vi "hmi-application.vi"() -> ()   [LabVIEW 2017]
doc: "Demonstrates how to write and receive CAN frames via the Network Interface on the same port. \n\nTo write and receive frames via the Network Interface:\n- select the CAN Network Interface (i.e. CAN0, CAN1, etc.)\n- select the Baud Rate\n- run the VI\n- press the write button to write frames to the can bus\n\nEnable RTR Button to send a Remote Transmission Request or to simply send an empty Frame to request an Answer Frame from a connected device.\n\nEnable Extended Button to write extended Identifier Format. This is done by setting the 30th bit to enable extended format with the driver."
uses:
  <vilib>/nican/nican.llb/ncNetAttr.ctl
panel:
  in  "Tab Control":enum32{"Program", "Settings"}(tab)
  in  "shutdown":bool
  in  "IND1":bool
  in  "IND2":bool
  in  "interface":string(combo)="CAN0" caption="Interface"
  # "PRESS AND HOLD"
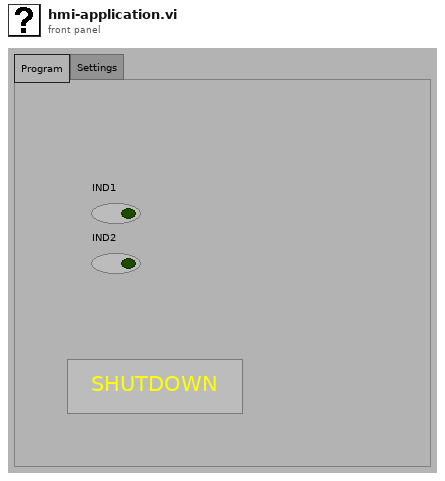
[diagram p1: front panel]
types:
  T1 = typedef "ncNetAttr.ctl" = cluster{"Start On Open":enum32{"FALSE", "TRUE"}, "Baud Rate":u32, "Read Queue Length":u32, "Write Queue Length":u32, "Standard Comparator":u32, "Standard Mask":u32, "Extended Comparator":u32, "Extended Mask":u32}
  T2 = typedef "xobjhandle.ctl" = u32
  T3 = typedef "CanFrameTimed.ctl" = cluster{"Timestamp":dbl, "ArbitrationId":u32, "IsRemote":u8, "DataLength":u8, "Data":u8[]}
  T4 = cluster{dbl, u32, "IsRemote":u8, "DataLength":u8, u8[]}
  T5 = cluster{dbl, u32, "IsRemote":u8, "DataLength":u8, u8[]}[]
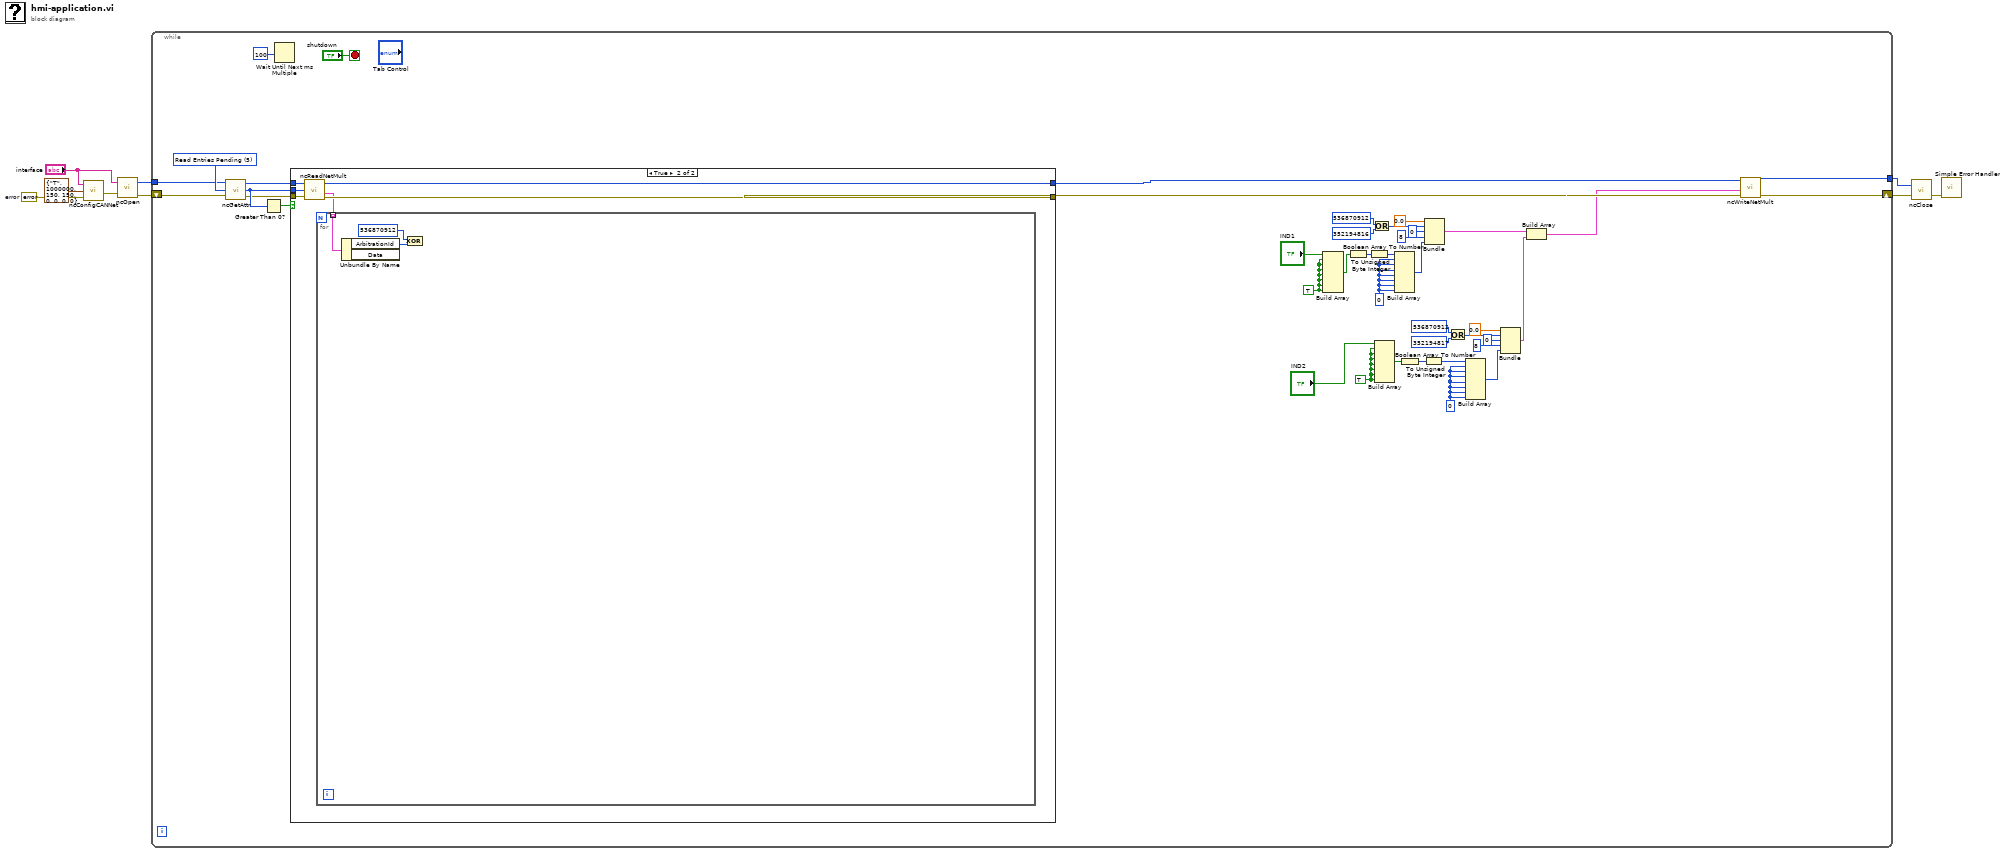
[diagram p0: block diagram]
diagram:
  w5 = errorcluster {"status"=FALSE, "code"=0, "source"=""}  # error
  n1 = call <vilib>:"ncConfigCANNet.vi"("Error in"=w5, "CAN Network Interface Config"=T1 {"Start On Open"=enum."TRUE", "Baud Rate"=1000000, "Read Queue Length"=150, "Write Queue Length"=150, "Standard Comparator"=0, "Standard Mask"=0, "Extended Comparator"=0, "Extended Mask"=0}, "ObjName"="interface") -> ("Error out"=w6:errorcluster)  [unwired: 2 in]
  n2 = call <vilib>:"ncOpen.vi"("Error in"=w6, "ObjName"="interface") -> ("Error out"=w9:errorcluster, "ObjHandle out"=w7:T2)
  n3 = while {
    tunnel: w7 -> [w40]
    tunnel: [w50] -> w2
    shift-right: [w51] -> w1
    shift-left: w9 -> [w39]
    stop <- "shutdown" stop-if-true
    w18 = TRUE ("element")
    w20 = TRUE ("element")
    w23 = u8 0
    w31 = u8 0
    w43 = u32 5 items=["(reserved)", "Protocol Version", "Software Version", "Object State", "(reserved)", "Read Entries Pending", "Write Entries Pending", "ReadMult Size for Notification", "Listen Only?", "Self Reception?", "Transmit Error Counter", "Receive Error Counter", "Single Shot Transmit?", "Series 2 Filter Mode", "Series 2 Mask", "Series 2 Comparator", "Serial Number", "Form Factor", "Series", "Transceiver Type", "Interface Number", "Series 2 Error/Arb Capture", "Transceiver Mode", "Transceiver External Outputs", "Transceiver External Inputs", "Start Trigger Behavior", "Log Comm Warnings", "User RTSI Frame", "Transmit Mode", "Log Start Trigger?", "Timestamp Format", "Master Timebase Rate", "Virtual Bus Timing"] ("AttrId")
    n4 = call <vilib>:"ncGetAttr.vi"("Error in"=w39, "AttrId"=w43, "ObjHandle in"=w40) -> ("Error out"=w44:errorcluster, "AttrValue"=w47:u32, "ObjHandle out"=w45:T2)
    n5 = Greater Than 0?(x=w47) -> (x > 0?=w46:bool)
    n6 = Wait Until Next ms Multiple(millisecond multiple=u32 100) -> ()  [unwired: 1 out]
    n7 = case shown="True" w46 {
      tunnel: [w52 w59] -> w41
      tunnel: [w53 w58] -> w42
      tunnel: w47 -> [_ w57]
      tunnel: w44 -> [w52 w56]
      tunnel: w45 -> [w53 w55]
      frame False {
      }
      frame True {
        n8 = call <vilib>:"ncReadNetMult.vi"("ObjHandle in"=w55, "Requested Number of Frames"=w57, "Error in"=w56) -> ("ObjHandle out"=w58:T2, "Data"=w54:T3[], "Error out"=w59:errorcluster)  [unwired: 1 out]
        n9 = for {
          tunnel: w54 -> [w62] mode=indexing
          n10 = Unbundle By Name(w62) -> ("ArbitrationId"=w60:u32)  [unwired: 1 out]
          n11 = Exclusive Or(1:w60, 2:u32 536870912 ("y")) -> ()  [unwired: 1 out]
        }
      }
    }
    n12 = Build Array("IND1", w20, w20, w20, w20, w20, w20, w20) -> (w14:bool[])
    n13 = Boolean Array To Number(Boolean array=w14) -> (number=w16:u32)
    n14 = To Unsigned Byte Integer(number=w16) -> (unsigned 8bit integer=w15:u8)
    n15 = Or(x=u32 536870912 ("y"), y=u32 352194816) -> (x .or. y?=w29:u32)
    n16 = Build Array("IND2", w18, w18, w18, w18, w18, w18, w18) -> (w19:bool[])
    n17 = Build Array(w15, w23, w23, w23, w23, w23, w23, w23) -> (w25:u8[])
    n18 = Boolean Array To Number(Boolean array=w19) -> (number=w12:u32)
    n19 = To Unsigned Byte Integer(number=w12) -> (unsigned 8bit integer=w13:u8)
    n20 = Bundle(0.0, w29, "IsRemote"=u8 0, "DataLength"=u8 8, w25) -> (w22:T4)  [unwired: 1 in]
    n21 = Or(x=u32 536870912 ("y"), y=u32 352194817) -> (x .or. y?=w37:u32)
    n22 = Build Array(w13, w31, w31, w31, w31, w31, w31, w31) -> (w33:u8[])
    n23 = Bundle(0.0, w37, "IsRemote"=u8 0, "DataLength"=u8 8, w33) -> (w11:T4)  [unwired: 1 in]
    n24 = Build Array(w22, w11) -> (w10:T5)
    n25 = call <vilib>:"ncWriteNetMult.vi"("Error in"=w41, "Data"=w10, "ObjHandle in"=w42) -> ("Error out"=w51:errorcluster, "ObjHandle out"=w50:T2)  [unwired: 7 in]
  }
  n26 = call <vilib>:"ncClose.vi"("Error in"=w1, "ObjHandle in"=w2) -> ("Error out"=w3:errorcluster)  [unwired: 1 in]
  n27 = call <vilib>:"Simple Error Handler.vi"("error in (no error)"=w3) -> ()  [unwired: 4 in, 5 out]
